vi "DriveDistanceAngle.vi"(0 "Distance":dbl=84.0, 1 "Drive Margin":dbl=12.0, 2 "Steer Margin":dbl=10.0, 5 "Angle":dbl=180.0, 7 "Starting Position":T1, 9 "Speed":dbl=0.5, 11 "error in":errorcluster, 12 "Start time":u32=1686895, 13 "Timeout (ms)":u32=5000) -> (4 "RobotDriveDevRef Out":T2={"DevStatus"={"status"=FALSE, "code"=0, "source"=""}, "Motors[]"=[{"DeviceStatus"={"status"=FALSE, "code"=0, "source"=""}, "Type"=enum."PWM", "PWM"={"Digital Module"=enum."Digital Module 1", "PWM Channel"=enum."PWM 2", "DeadBand"={"Name"="Victor", "maxPositivePwm"=208, "minPositivePwm"=129, "centerPwm"=128, "maxNegativePwm"=127, "minNegativePwm"=54, "angularRange"=0}}, "CAN"={"Device Number"=0, "Control Mode"=enum."Percent VBus", "Semaphore"=refnum, "Max Vout"=0.0}, "Invert"=FALSE, "TransformRef"=refnum, "InvTransformRef"=refnum}, {"DeviceStatus"={"status"=FALSE, "code"=0, "source"=""}, "Type"=enum."PWM", "PWM"={"Digital Module"=enum."Digital Module 1", "PWM Channel"=enum."PWM 1", "DeadBand"={"Name"="Victor", "maxPositivePwm"=208, "minPositivePwm"=129, "centerPwm"=128, "maxNegativePwm"=127, "minNegativePwm"=54, "angularRange"=0}}, "CAN"={"Device Number"=0, "Control Mode"=enum."Percent VBus", "Semaphore"=refnum, "Max Vout"=0.0}, "Invert"=TRUE, "TransformRef"=refnum, "InvTransformRef"=refnum}, {"DeviceStatus"={"status"=FALSE, "code"=0, "source"=""}, "Type"=enum."PWM", "PWM"={"Digital Module"=enum."Digital Module 1", "PWM Channel"=enum."PWM 4", "DeadBand"={"Name"="Victor", "maxPositivePwm"=208, "minPositivePwm"=129, "centerPwm"=128, "maxNegativePwm"=127, "minNegativePwm"=54, "angularRange"=0}}, "CAN"={"Device Number"=0, "Control Mode"=enum."Percent VBus", "Semaphore"=refnum, "Max Vout"=0.0}, "Invert"=FALSE, "TransformRef"=refnum, "InvTransformRef"=refnum}, {"DeviceStatus"={"status"=FALSE, "code"=0, "source"=""}, "Type"=enum."PWM", "PWM"={"Digital Module"=enum."Digital Module 1", "PWM Channel"=enum."PWM 3", "DeadBand"={"Name"="Victor", "maxPositivePwm"=208, "minPositivePwm"=129, "centerPwm"=128, "maxNegativePwm"=127, "minNegativePwm"=54, "angularRange"=0}}, "CAN"={"Device Number"=0, "Control Mode"=enum."Percent VBus", "Semaphore"=refnum, "Max Vout"=0.0}, "Invert"=TRUE, "TransformRef"=refnum, "InvTransformRef"=refnum}, {"DeviceStatus"={"status"=FALSE, "code"=0, "source"=""}, "Type"=enum."PWM", "PWM"={"Digital Module"=enum."Digital Module 1", "PWM Channel"=enum."PWM 6", "DeadBand"={"Name"="Victor", "maxPositivePwm"=208, "minPositivePwm"=129, "centerPwm"=128, "maxNegativePwm"=127, "minNegativePwm"=54, "angularRange"=0}}, "CAN"={"Device Number"=0, "Control Mode"=enum."Percent VBus", "Semaphore"=refnum, "Max Vout"=0.0}, "Invert"=FALSE, "TransformRef"=refnum, "InvTransformRef"=refnum}, {"DeviceStatus"={"status"=FALSE, "code"=0, "source"=""}, "Type"=enum."PWM", "PWM"={"Digital Module"=enum."Digital Module 1", "PWM Channel"=enum."PWM 5", "DeadBand"={"Name"="Victor", "maxPositivePwm"=208, "minPositivePwm"=129, "centerPwm"=128, "maxNegativePwm"=127, "minNegativePwm"=54, "angularRange"=0}}, "CAN"={"Device Number"=0, "Control Mode"=enum."Percent VBus", "Semaphore"=refnum, "Max Vout"=0.0}, "Invert"=TRUE, "TransformRef"=refnum, "InvTransformRef"=refnum}], "Square Inputs"=TRUE, "Max Output"=1.0, "Isochronous"=FALSE}, 6 "At Target":bool=TRUE, 8 "Timeout?":bool, 15 "error out":errorcluster)   [LabVIEW 2013]
uses:
  <vilib>/Rock Robotics/WPI/RobotDrive/WPI_RobotDriveDevRef.ctl
  <vilib>/Rock Robotics/WPI/MotorControl/WPI_MotorControlDeviceRef.ctl
  <vilib>/Rock Robotics/SystemInterfaces/Typedef/FPGA_TypedefDigitalModule.ctl
  <vilib>/Rock Robotics/SystemInterfaces/DIO/FPGA_DIOPWMChannel.ctl
  <vilib>/Rock Robotics/WPI/PWM/WPI_PWMDeadband.ctl
  <vilib>/Rock Robotics/WPI/CAN/Jaguar/SubVIs/WPI_CANJaguar_ControlMode.ctl
  <vilib>/Rock Robotics/WPI/PWM/WPI_PWMTransform_ConPane.ctl
  Position Typedef.ctl
  Robot Global Data.vi
  <vilib>/Rock Robotics/WPI/RobotDrive/WPI_RobotDriveGetSetRefNum.vi
  <vilib>/addons/control/pid/NI_PID_pid.lvlib
panel:
  in  "Drive PID gains":T10={"proportional gain (Kc)"=0.12, "integral time (Ti, min)"=0.0, "derivative time (Td, min)"=0.0} {"derivative time (Td, min)" format="%.3f"; "integral time (Ti, min)" format="%.3f"; "proportional gain (Kc)" format="%.3f"}
  in  "Steer PID gains":T10={"proportional gain (Kc)"=0.0005, "integral time (Ti, min)"=0.0, "derivative time (Td, min)"=0.0} {"derivative time (Td, min)" format="%#.7g"; "integral time (Ti, min)" format="%#.6g"; "proportional gain (Kc)" format="%#.6g"}
  in  "Steering Saturation":dbl=1.0
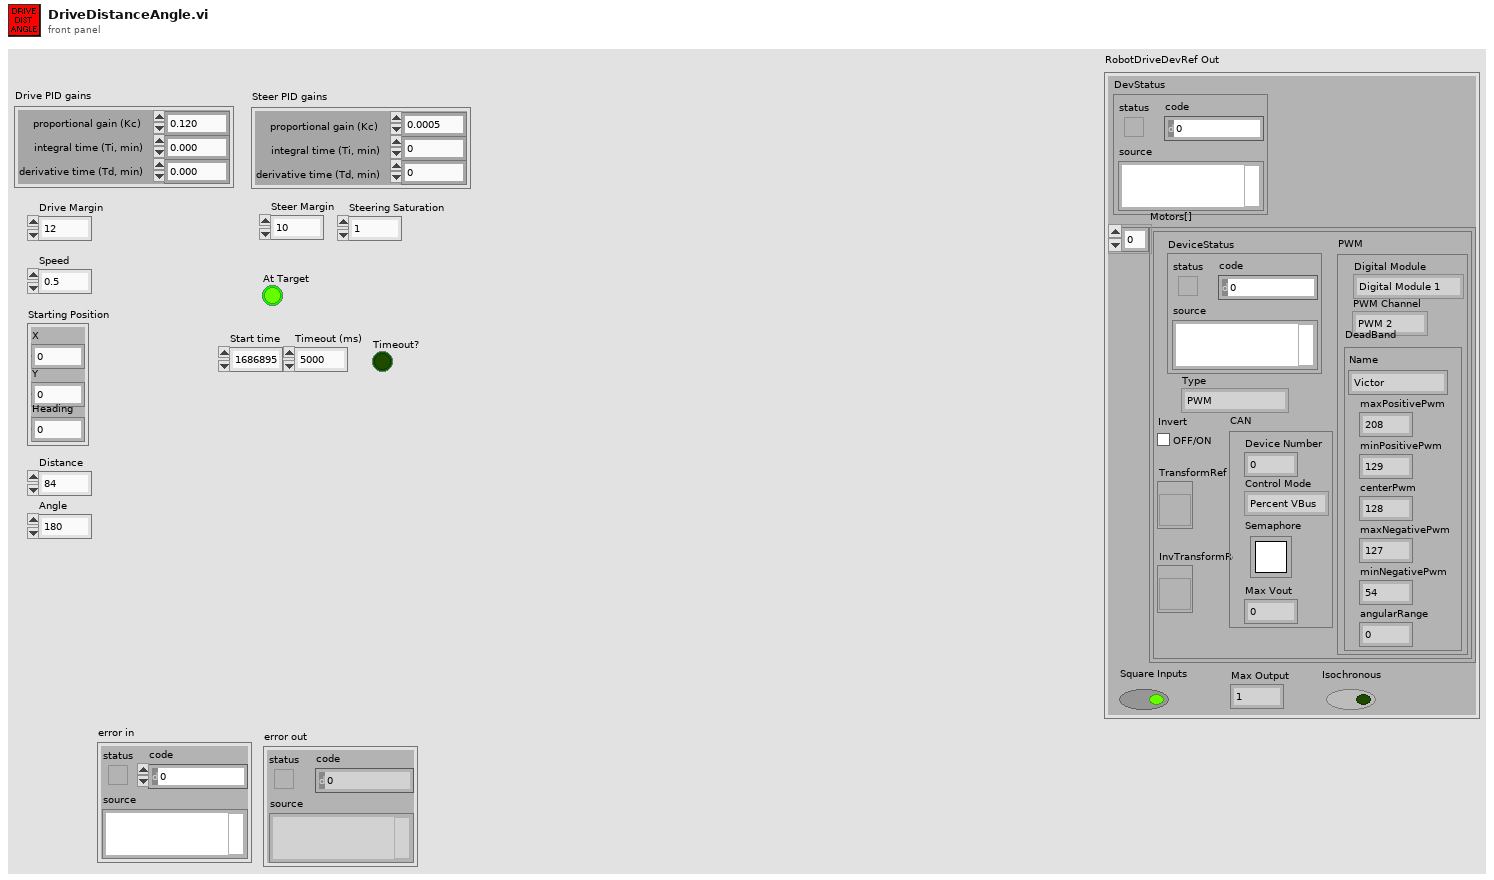
[diagram p1: front panel]
types:
  T1 = typedef "Position Typedef.ctl" = cluster{"X":dbl, "Y":dbl, "Heading":dbl}
  T2 = typedef "WPI_RobotDriveDevRef.ctl" = cluster{"DevStatus":errorcluster, "Motors[]":T3[], "Square Inputs":bool, "Max Output":dbl, "Isochronous":bool}
  T3 = typedef "WPI_MotorControlDeviceRef.ctl" = cluster{"DeviceStatus":errorcluster, "Type":enum16{"PWM", "CAN"}, "PWM":cluster{"Digital Module":T4, "PWM Channel":T5, "DeadBand":T6}, "CAN":cluster{"Device Number":u8, "Control Mode":T7, "Semaphore":T8, "Max Vout":dbl}, "Invert":bool, "TransformRef":T9, "InvTransformRef":T9}
  T4 = typedef "FPGA_TypedefDigitalModule.ctl" = enum16{"Digital Module 1", "Digital Module 2"}
  T5 = typedef "FPGA_DIOPWMChannel.ctl" = enum8{"PWM 1", "PWM 2", "PWM 3", "PWM 4", "PWM 5", "PWM 6", "PWM 7", "PWM 8", "PWM 9", "PWM 10", "Invalid"}
  T6 = typedef "WPI_PWMDeadband.ctl" = cluster{"Name":string, "maxPositivePwm":i32, "minPositivePwm":i32, "centerPwm":i32, "maxNegativePwm":i32, "minNegativePwm":i32, "angularRange":u16}
  T7 = typedef "WPI_CANJaguar_ControlMode.ctl" = enum8{"Percent VBus", "Current", "Speed", "Position", "Voltage"}
  T8 = typedef "Semaphore RefNum" = refnum<k1>
  T9 = typedef "WPI_PWMTransform_ConPane.ctl" = refnum<vi>
  T10 = cluster{"proportional gain (Kc)":dbl, "integral time (Ti, min)":dbl, "derivative time (Td, min)":dbl}
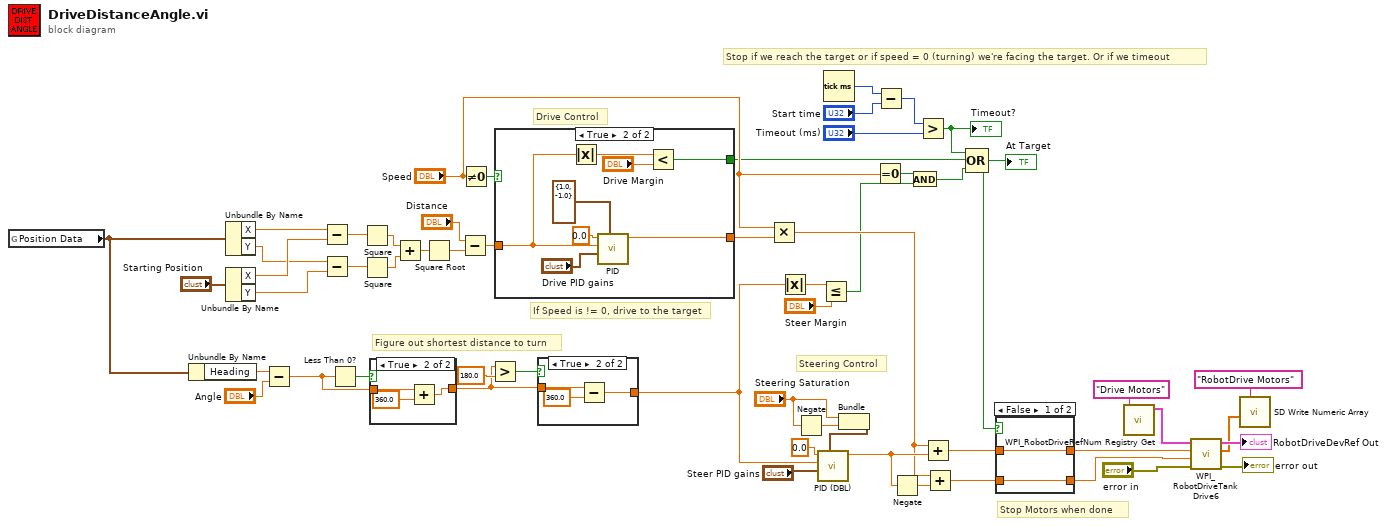
[diagram p0: block diagram]
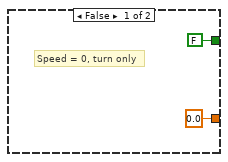
[diagram p5: hidden frame]
diagram:
  # "Stop Motors when done"
  # "Figure out shortest distance to turn"
  # "Stop if we reach the target or if speed = 0 (turning) we're facing the target. Or if we timeout"
  # "Drive Control"
  # "If Speed is != 0, drive to the target"
  # "Steering Control"
  n1 = global read "Robot Global Data.vi" "Position Data"() -> (w9:T1)
  n2 = Unbundle By Name(w9) -> ("Heading"=w8:dbl)
  n3 = Unbundle By Name(w9) -> ("X"=w21:dbl, "Y"=w19:dbl)
  n4 = Unbundle By Name("Starting Position") -> ("X"=w20:dbl, "Y"=w18:dbl)
  n5 = Subtract(x=w8, y="Angle") -> (x-y=w2:dbl)
  n6 = Subtract(x=w21, y=w20) -> (x-y=w14:dbl)
  n7 = Subtract(x=w19, y=w18) -> (x-y=w13:dbl)
  n8 = Less Than 0?(x=w2) -> (x < 0?=w4:bool)
  n9 = Square(x=w14) -> (x^2=w15:dbl)
  n10 = Square(x=w13) -> (x^2=w16:dbl)
  n11 = case shown="True" w4 {
    tunnel: w2 -> [w57 w59]
    tunnel: [w57 w58] -> w3
    frame False {
    }
    frame True {
      n12 = Add(x=w59, y=360.0) -> (x+y=w58:dbl)
    }
  }
  n13 = Add(x=w15, y=w16) -> (x+y=w17:dbl)
  n14 = Square Root(x=w17) -> (sqrt(x)=w12:dbl)
  n15 = Subtract(x="Distance", y=w12) -> (x-y=w10:dbl)
  n16 = Not Equal To 0?(x="Speed") -> (x != 0?=w49:bool)
  n17 = Greater?(x=w3, y=180.0) -> (0:w5:bool)
  n18 = case shown="True" w49 {
    tunnel: [FALSE w65] -> w43
    tunnel: [0.0 ("output") w64] -> w48
    tunnel: w10 -> [_ w63]
    frame False {
      # "Speed = 0, turn only"
    }
    frame True {
      n19 = Absolute Value(x=w63) -> (abs(x)=w68:dbl)
      n20 = call-poly <vilib>:"PID.vi"("output range"=cluster{"output high":dbl, "output low":dbl} {"output high"=1.0, "output low"=-1.0}, "PID gains"="Drive PID gains", "process variable"=w63, "setpoint"=0.0 ("y")) -> ("output"=w64:dbl)  [unwired: 2 in, 5 out]
      n21 = Less?(x=w68, y="Drive Margin") -> (x < y?=w65:bool)
    }
  }
  n22 = case shown="True" w5 {
    tunnel: w3 -> [w71 w74]
    tunnel: [w71 w73] -> w1
    frame False {
    }
    frame True {
      n23 = Subtract(x=w74, y=360.0) -> (x-y=w73:dbl)
    }
  }
  n24 = Multiply(x="Speed", y=w48) -> (x*y=w45:dbl)
  n25 = Absolute Value(x=w1) -> (abs(x)=w51:dbl)
  n26 = Negate(x="Steering Saturation") -> (-x=w55:dbl)
  n27 = Less Or Equal?(x=w51, y="Steer Margin") -> (x <= y?=w40:bool)
  n28 = Tick Count (ms)() -> (millisecond timer value=w32:u32)
  n29 = Bundle("Steering Saturation"="Steering Saturation", w55) -> (w54:cluster{"Steering Saturation":dbl, dbl})  [unwired: 1 out]
  n30 = call <vilib>:"PID (DBL).vi"("output range"=w54, "PID gains"="Steer PID gains", "process variable"=w1, "setpoint"=0.0) -> ("output"=w47:dbl)  [unwired: 2 in, 5 out]
  n31 = Equal To 0?(x="Speed") -> (x = 0?=w41:bool)
  n32 = Subtract(x=w32, y="Start time") -> (x-y=w31:u32)
  n33 = Negate(x=w47) -> (-x=w46:dbl)
  n34 = And(x=w41, y=w40) -> (x .and. y?=w42:bool)
  n35 = Greater?(x=w31, y="Timeout (ms)") -> (0:w28:bool)
  "Timeout?" <- w28
  n36 = Add(x=w45, y=w47) -> (x+y=w26:dbl)
  n37 = Add(x=w45, y=w46) -> (x+y=w25:dbl)
  n38 = Compound Arithmetic op=OR(w28, w43, w42) -> (w27:bool)
  "At Target" <- w27
  n39 = case shown="False" w27 {
    tunnel: w26 -> [w76 w78]
    tunnel: w25 -> [w75 w77]
    tunnel: [w76 w78] -> w24
    tunnel: [w75 w77] -> w23
    frame False {
    }
    frame True {
    }
  }
  n40 = call <vilib>:"WPI_RobotDriveRefNum Registry Get.vi"("refnum name"="Drive Motors") -> ("RobotDriveDevRef"=w37:T2)  [unwired: 1 in, 9 out]
  n41 = call "WPI_RobotDriveTankDrive6.vi"("error in (no error)"="error in", "Right axis value"=w23, "Left axis value"=w24, "RobotDriveDevRef"=w37) -> ("error out"=→"error out":errorcluster, "Motor Values"=w33:dbl[], "RobotDriveDevRef"=→"RobotDriveDevRef Out":T2)  [unwired: 5 in]
  n42 = call <vilib>:"SD Write Numeric Array.vi"("Numeric Array"=w33, "Name"="RobotDrive Motors") -> ()  [unwired: 8 in, 2 out]
